vi "capex chamber control.vi"(11 "Which chamber":enum16{"Little chamber", "Big chamber"}(ring)) -> ()   [LabVIEW 2013]
panel:
  in  "stop":bool
  out "String":string
  out "Humidity process value":dbl caption="Process value"
  in  "Humidity setpoint":dbl caption="Setpoint"
  out "Temperature process value":dbl caption="Process value"
  in  "Temperature setpoint":dbl caption="Setpoint"
  # "Temperature"
  # "10-45C"
  # "Humidity"
  # "0-100%"
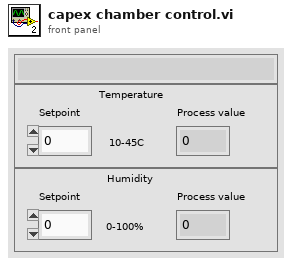
[diagram p1: front panel]
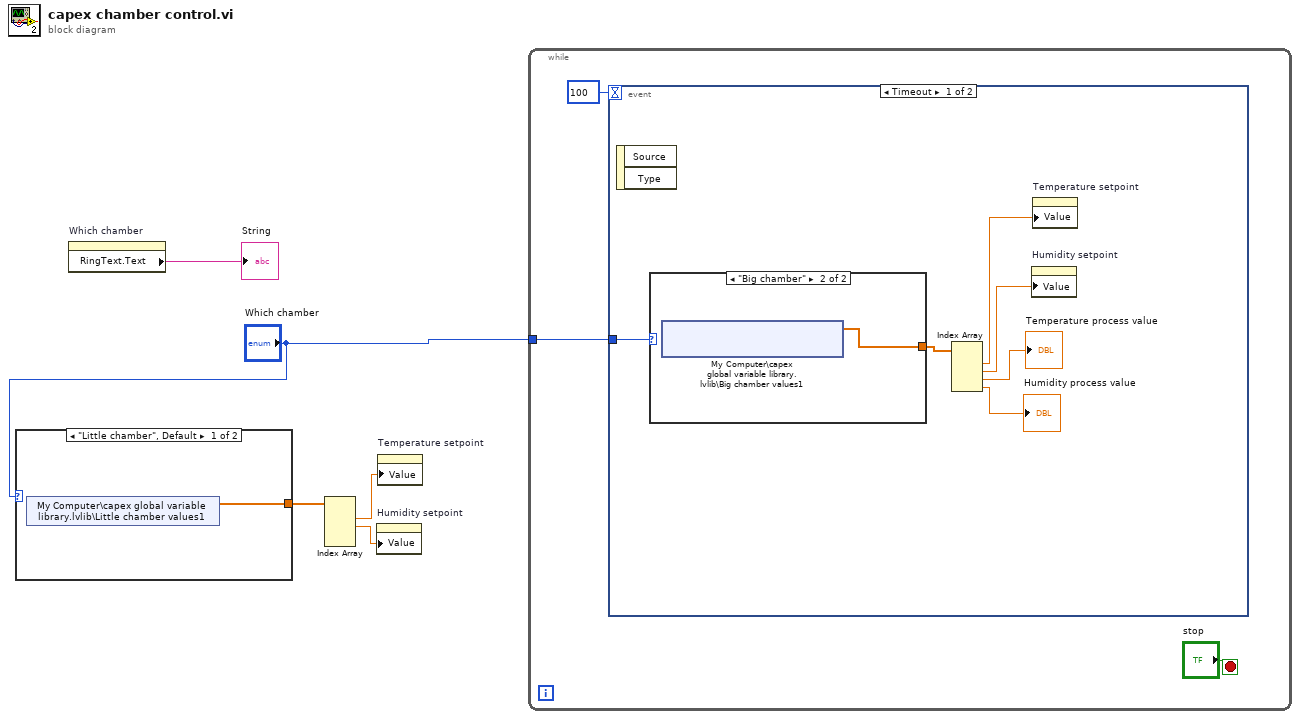
[diagram p0: block diagram]
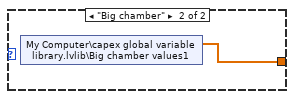
[diagram p2: hidden frame]
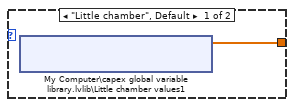
[diagram p3: hidden frame]
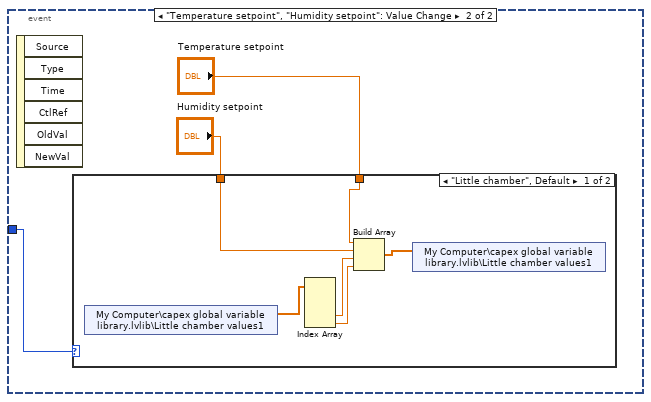
[diagram p4: hidden frame]
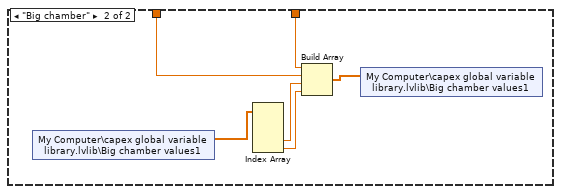
[diagram p5: hidden frame]
diagram:
  n1 = case shown="\"Little chamber\", Default" "Which chamber" {
    tunnel: [w6 w7] -> w2
    frame "Little chamber", Default {
      n2 = shared-variable "My Computer\\capex global variable library.lvlib\\Little chamber values1"() -> (w6:dbl[])  [unwired: 1 in, 1 out]
    }
    frame "Big chamber" {
      n3 = shared-variable "My Computer\\capex global variable library.lvlib\\Big chamber values1"() -> (w7:dbl[])  [unwired: 1 in, 1 out]
    }
  }
  n4 = property on="Which chamber" class="Enum (strict)"() -> ("RingText.Text"=→"String":string)  [unwired: 2 in, 2 out]
  n5 = Index Array(array=w2) -> (element #1=w4:dbl, element #2=w3:dbl)  [unwired: 4 in, 2 out]
  n6 = property on="Humidity setpoint" class="DigNum (strict)"("Value"=w3) -> ()  [unwired: 2 in, 2 out]
  n7 = property on="Temperature setpoint" class="DigNum (strict)"("Value"=w4) -> ()  [unwired: 2 in, 2 out]
  n8 = while {
    tunnel: "Which chamber" -> [w9]
    stop <- "stop" stop-if-true
    n9 = event shown="[0] Timeout" {
      selector: _ -> [_ _]
      dyn-events: _ -> [_ _]
      timeout: 100 -> [_ _]
      tunnel: w9 -> [w14 w21]
      event Timeout {
        n10 = event-data() -> ()  [unwired: 1 in, 2 out]
        n11 = case shown="\"Big chamber\"" w14 {
          tunnel: [w17 w18] -> w13
          frame "Little chamber", Default {
            n12 = shared-variable "My Computer\\capex global variable library.lvlib\\Little chamber values1"() -> (w17:dbl[])  [unwired: 1 in, 2 out]
          }
          frame "Big chamber" {
            n13 = shared-variable "My Computer\\capex global variable library.lvlib\\Big chamber values1"() -> (w18:dbl[])  [unwired: 1 in, 2 out]
          }
        }
        n14 = Index Array(array=w13) -> (element #1=w12:dbl, element #2=w11:dbl, element #3=→"Temperature process value":dbl, element #4=→"Humidity process value":dbl)  [unwired: 4 in]
        n15 = property on="Humidity setpoint" class="DigNum (strict)"("Value"=w11) -> ()  [unwired: 2 in, 2 out]
        n16 = property on="Temperature setpoint" class="DigNum (strict)"("Value"=w12) -> ()  [unwired: 2 in, 2 out]
      }
      event "Temperature setpoint", "Humidity setpoint": Value Change {
        n17 = event-data() -> ()  [unwired: 1 in, 6 out]
        n18 = case shown="\"Little chamber\", Default" w21 {
          tunnel: "Temperature setpoint" -> [w23 w30]
          tunnel: "Humidity setpoint" -> [w22 w29]
          frame "Little chamber", Default {
            n19 = shared-variable "My Computer\\capex global variable library.lvlib\\Little chamber values1"() -> (w27:dbl[])  [unwired: 1 in, 1 out]
            n20 = Index Array(array=w27) -> (element #3=w26:dbl, element #4=w25:dbl)  [unwired: 4 in, 2 out]
            n21 = Build Array(w23, w22, w26, w25) -> (w24:dbl[])
            n22 = shared-variable "My Computer\\capex global variable library.lvlib\\Little chamber values1"(w24) -> ()  [unwired: 1 in, 1 out]
          }
          frame "Big chamber" {
            n23 = shared-variable "My Computer\\capex global variable library.lvlib\\Big chamber values1"() -> (w33:dbl[])  [unwired: 1 in, 1 out]
            n24 = Index Array(array=w33) -> (element #3=w32:dbl, element #4=w31:dbl)  [unwired: 4 in, 2 out]
            n25 = Build Array(w30, w29, w32, w31) -> (w28:dbl[])
            n26 = shared-variable "My Computer\\capex global variable library.lvlib\\Big chamber values1"(w28) -> ()  [unwired: 1 in, 1 out]
          }
        }
      }
    }
  }
